vi "GetChosenDeviceByName.vi"(1 "Chosen Name":string) -> (0 "Device Out":refnum<class "Device.lvclass">)   [LabVIEW 2013]
uses:
  Device/Device.lvclass
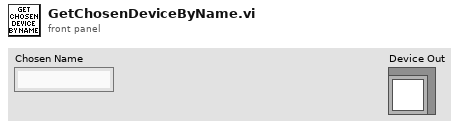
[diagram p1: front panel]
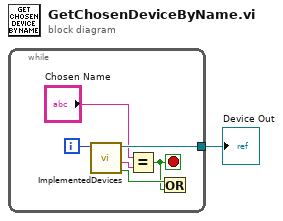
[diagram p0: block diagram]
diagram:
  n1 = while {
    tunnel: [w7] -> w1
    i -> [w2]
    stop <- w5 stop-if-true
    n2 = call "ImplementedDevices.vi"("Index"=w2) -> ("Not In List"=w6:bool, "Menu Name"=w4:string, "Device Out"=w7:refnum<class "Device.lvclass">)  [unwired: 8 in]
    n3 = Equal?(x="Chosen Name", y=w4) -> (x = y?=w5:bool)
    n4 = Or(x=w6, y=w5) -> ()  [unwired: 1 out]
  }
  "Device Out" <- w1
